vi "Dosimetric Threshold Probablities.vi"(2 "Standard Deviation [Gy]":dbl=1.0, 3 "Estimated Dose [Gy]":dbl, 4 "Decision Threshold [Gy]":dbl) -> (0 "% Probability Below Threshold":dbl=0.5 format="%#.2g", 1 "% Probability Above Threshold":dbl=0.5 format="%#.2g")   [LabVIEW 2016]
uses:
  <vilib>/gmath/statdist.llb/Normal CDF.vi
  <vilib>/gmath/NI_Gmath.lvlib
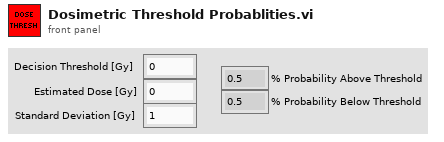
[diagram p1: front panel]
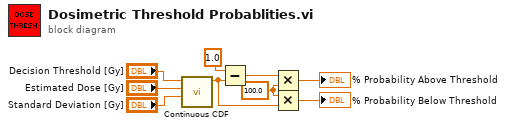
[diagram p0: block diagram]
diagram:
  w5 = 100.0 ("x")
  n1 = call-poly <vilib>:"Continuous CDF.vi"("std"="Standard Deviation [Gy]", "mean"="Estimated Dose [Gy]", "x"="Decision Threshold [Gy]") -> ("cdf(x)"=w4:dbl)  [unwired: 7 in, 1 out]
  n2 = Subtract(x=1.0, y=w4) -> (x-y=w3:dbl)
  n3 = Multiply(x=w3, y=w5) -> (x*y=→"% Probability Above Threshold":dbl)
  n4 = Multiply(x=w5, y=w4) -> (x*y=→"% Probability Below Threshold":dbl)
